vi "Helper - Rounding Direction Chooser.vi"(6 "Buoy\nSide":enum16{"Starboard", "Port"}(ring), 8 "Point NORTH 2":dbl, 9 "Point EAST 2":dbl, 10 "Point NORTH":dbl, 11 "Point EAST":dbl) -> (0 "End Point NORTH":dbl, 1 "End Point EAST":dbl, 2 "Start Point NORTH":dbl, 3 "Start Point EAST":dbl)   [LabVIEW 2011]
doc: "This VI takes two previously created waypoints as input. Depending on the state of the ENUM variable (Starboard or Port) the attributes STARTPOINT and ENDPOINT are assigned to the two points."
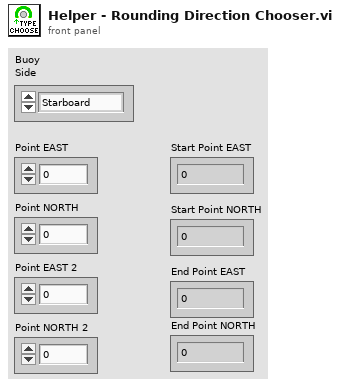
[diagram p1: front panel]
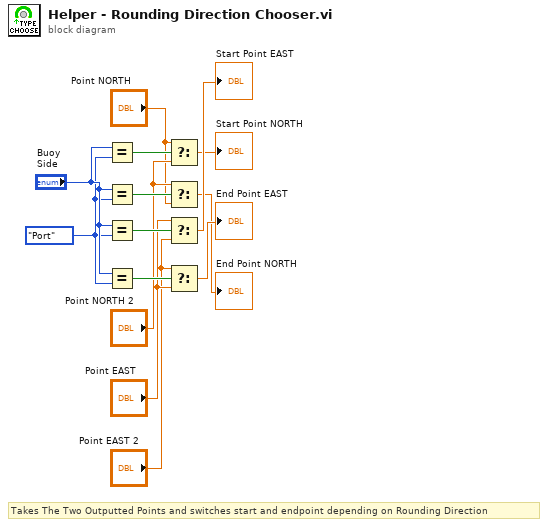
[diagram p0: block diagram]
diagram:
  w1 = enum16{"Starboard", "Port"}."Port" ("y")
  # "Takes The Two Outputted Points and switches start and endpoint depending on Rounding Direction"
  n1 = Equal?(x="Buoy\nSide", y=w1) -> (x = y?=w14:bool)
  n2 = Equal?(x="Buoy\nSide", y=w1) -> (x = y?=w10:bool)
  n3 = Equal?(x="Buoy\nSide", y=w1) -> (x = y?=w13:bool)
  n4 = Equal?(x="Buoy\nSide", y=w1) -> (x = y?=w9:bool)
  n5 = Select(t="Point NORTH", s=w14, f="Point NORTH 2") -> (s? t:f=→"Start Point NORTH":dbl)
  n6 = Select(t="Point NORTH 2", s=w10, f="Point NORTH") -> (s? t:f=→"End Point NORTH":dbl)
  n7 = Select(t="Point EAST", s=w13, f="Point EAST 2") -> (s? t:f=→"Start Point EAST":dbl)
  n8 = Select(t="Point EAST 2", s=w9, f="Point EAST") -> (s? t:f=→"End Point EAST":dbl)
